vi "Tosca-Plot AI Data.vi"(0 "state in":T2, 5 "Data":cluster{dbl[][], "DI":bool[][]}, 11 "error in (no error)":errorcluster, 12 "Analog":refnum<vi>, 13 "Controls":T1) -> (4 "state out":T2, 15 "error out":errorcluster)   [LabVIEW 2020]
uses:
  Typedefs/Tosca-AI Plot State.ctl
  Typedefs/Tosca-AI Live Controls.ctl
  epl-vi-lib/Utility VIs/Array Manipulation VIs/Array-Dimensions (2D).vi
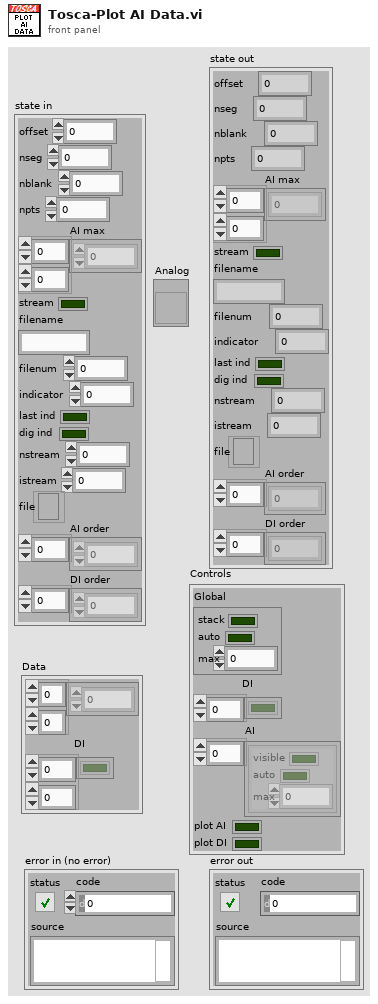
[diagram p1: front panel]
types:
  T1 = typedef "Tosca-AI Live Controls.ctl" = cluster{"Global":cluster{"stack":bool, "auto":bool, "max":dbl}, "DI":bool[], "AI":cluster{"visible":bool, "auto":bool, "max":dbl}[], "plot AI":bool, "plot DI":bool}
  T2 = typedef "Tosca-AI Plot State.ctl" = cluster{"offset":i32, "nseg":i32, "nblank":i32, "npts":i32, "AI max":dbl[][], "stream":bool, "filename":string, "filenum":i32, "indicator":i32, "last ind":bool, "dig ind":bool, "nstream":i32, "istream":i32, "file":refnum<file>, "AI order":i32[], "DI order":i32[]}
  T3 = cluster{"visible":bool, "auto":bool, "max":dbl}[]
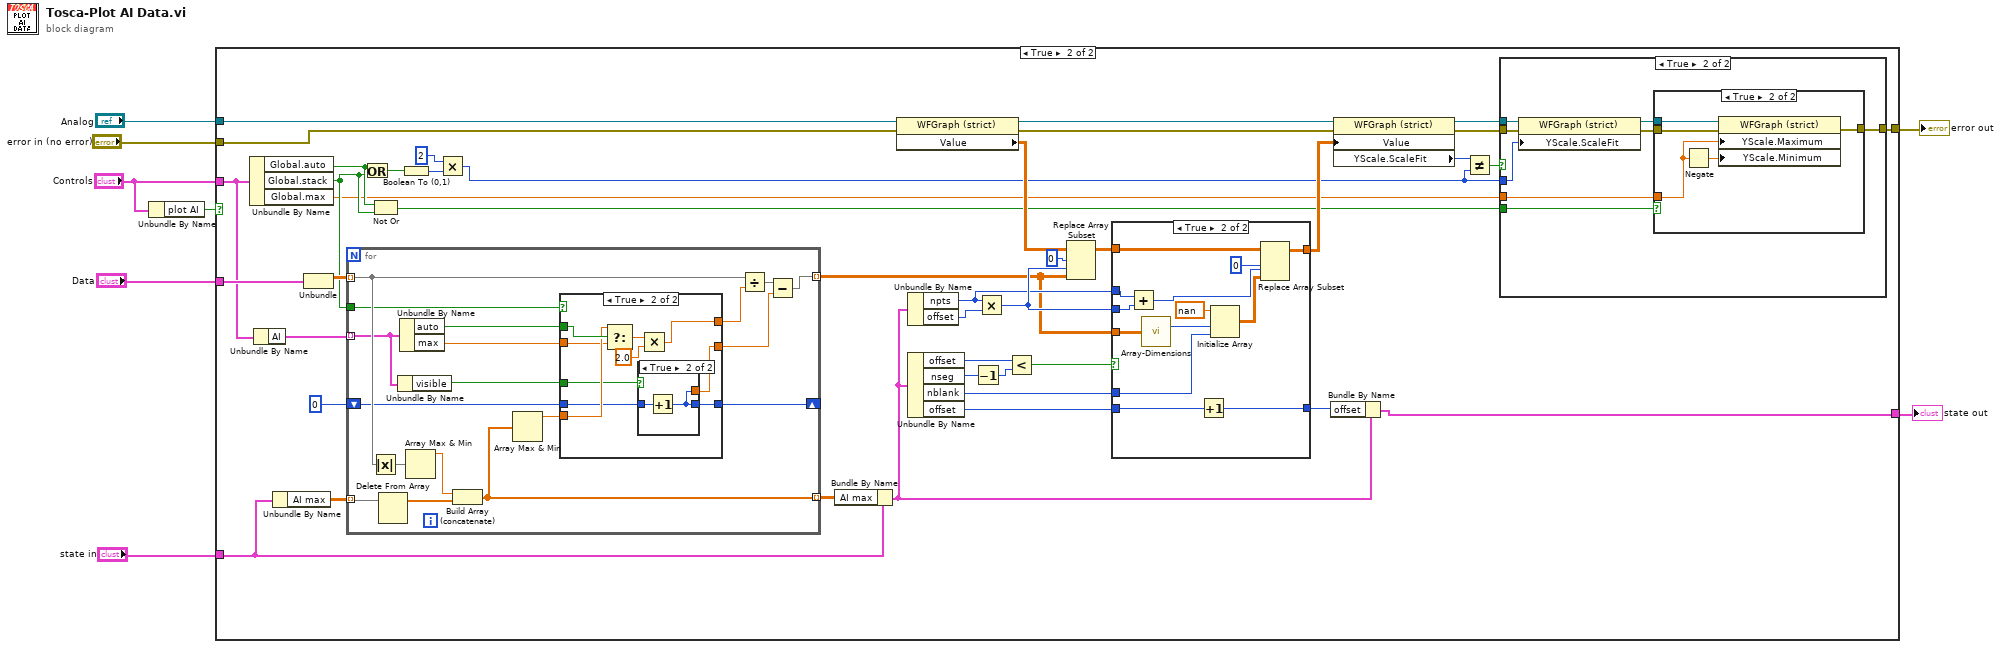
[diagram p0: block diagram]
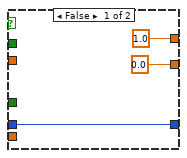
[diagram p5: hidden frame]
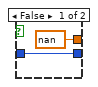
[diagram p6: hidden frame]
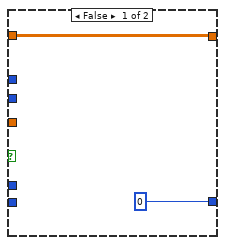
[diagram p7: hidden frame]
diagram:
  n1 = Unbundle By Name("Controls") -> ("plot AI"=w2:bool)
  n2 = case shown="True" w2 {
    tunnel: "Analog" -> [_ w52]
    tunnel: "error in (no error)" -> [w10 w51]
    tunnel: "Data" -> [_ w50]
    tunnel: "state in" -> [w9 w31]
    tunnel: "Controls" -> [_ w26]
    tunnel: [w10 w14] -> w4
    tunnel: [w9 w11] -> w1
    frame False {
    }
    frame True {
      n3 = Unbundle By Name(w26) -> ("Global.auto"=w21:bool, "Global.stack"=w20:bool, "Global.max"=w12:dbl)
      n4 = Unbundle By Name(w26) -> ("AI"=w27:T3)
      n5 = Unbundle By Name(w31) -> ("AI max"=w30:dbl[][])
      n6 = Unbundle(w50) -> (w33:dbl[][])  [unwired: 1 out]
      n7 = for {
        tunnel: w33 -> [w84] mode=indexing
        tunnel: [w85] -> w32 mode=indexing
        tunnel: w30 -> [w82] mode=indexing
        tunnel: [w78] -> w28 mode=indexing
        tunnel: w20 -> [w75]
        tunnel: w27 -> [w69] mode=indexing
        shift-right: [w76] -> _
        shift-left: 0 -> [w77]
        n8 = Absolute Value(x=w84) -> (abs(x)=w83:dbl[])
        n9 = Delete From Array(array=w82) -> (array with subset deleted=w80:dbl[])  [unwired: 2 in, 1 out]
        n10 = Unbundle By Name(w69) -> ("visible"=w68:bool)
        n11 = Unbundle By Name(w69) -> ("auto"=w72:bool, "max"=w70:dbl)
        n12 = Array Max & Min(array=w83) -> (max value=w79:dbl)  [unwired: 3 out]
        n13 = Build Array (concatenate)(w79, w80) -> (w78:dbl[])
        n14 = Array Max & Min(array=w78) -> (max value=w71:dbl)  [unwired: 3 out]
        n15 = case shown="True" w75 {
          tunnel: w77 -> [w87 w91]
          tunnel: [w87 w90] -> w76
          tunnel: [1.0 w93] -> w74
          tunnel: [0.0 w89] -> w73
          tunnel: w72 -> [_ w98]
          tunnel: w71 -> [_ w97]
          tunnel: w70 -> [_ w96]
          tunnel: w68 -> [_ w92]
          frame False {
          }
          frame True {
            n16 = Select(t=w97, s=w98, f=w96) -> (s? t:f=w95:dbl)
            n17 = case shown="True" w92 {
              tunnel: w91 -> [w100 w102]
              tunnel: [w100 w101] -> w90
              tunnel: [nan w101] -> w89
              frame False {
              }
              frame True {
                n18 = Increment(x=w102) -> (x+1=w101:i32)
              }
            }
            n19 = Multiply(x=w95, y=2.0) -> (x*y=w93:dbl)
          }
        }
        n20 = Divide(x=w84, y=w74) -> (x/y=w81:dbl[])
        n21 = Subtract(x=w81, y=w73) -> (x-y=w85:dbl[])
      }
      n22 = Or(x=w21, y=w20) -> (x .or. y?=w25:bool)
      n23 = Not Or(1:w20, 2:w21) -> (0:w13:bool)
      n24 = Boolean To (0,1)(Boolean=w25) -> (0, 1=w24:i16)
      n25 = Multiply(x=i16 2 ("y"), y=w24) -> (x*y=w15:i16)
      n26 = Bundle By Name(cluster=w31, "AI max"=w28) -> (w29:T2)
      n27 = property class="WFGraph (strict)"(reference=w52, error in=w51) -> (reference out=w47:refnum<vi>, error out=w46:errorcluster, "Value"=w49:dbl[][])
      n28 = Unbundle By Name(w29) -> ("npts"=w37:i32, "offset"=w45:i32)
      n29 = Unbundle By Name(w29) -> ("offset"=w44:i32, "nseg"=w43:i32, "nblank"=w41:i32, "offset"=w35:i32)
      n30 = Decrement(x=w43) -> (x-1=w42:i32)
      n31 = Multiply(x=w37, y=w45) -> (x*y=w38:i32)
      n32 = Less?(x=w44, y=w42) -> (x < y?=w39:bool)
      n33 = Replace Array Subset(array=w49, new element=w32, index (row)=0 ("disabled index (row)"), index (col)=w38) -> (w40:dbl[][])
      n34 = case shown="True" w39 {
        tunnel: w32 -> [_ w117]
        tunnel: w41 -> [_ w115]
        tunnel: w40 -> [w104 w113]
        tunnel: w38 -> [_ w110]
        tunnel: w37 -> [_ w109]
        tunnel: [w104 w107] -> w36
        tunnel: w35 -> [_ w106]
        tunnel: [0 w105] -> w34
        frame False {
        }
        frame True {
          n35 = Add(x=w109, y=w110) -> (x+y=w108:i32)
          n36 = call-poly "Array-Dimensions.vi"("2D Array"=w117) -> ("# rows"=w116:i32)  [unwired: 13 in, 1 out]
          n37 = Increment(x=w106) -> (x+1=w105:i32)
          n38 = Initialize Array(nan, w116, w115) -> (w112:dbl[][])
          n39 = Replace Array Subset(array=w113, new element=w112, index (row)=0, index (col)=w108) -> (w107:dbl[][])
        }
      }
      n40 = Bundle By Name(cluster=w29, "offset"=w34) -> (w11:T2)
      n41 = property class="WFGraph (strict)"(reference=w47, error in=w46, "Value"=w36) -> (reference out=w19:refnum<vi>, error out=w18:errorcluster, "YScale.ScaleFit"=w17:u8)
      n42 = Not Equal?(x=w17, y=w15) -> (x != y?=w16:bool)
      n43 = case shown="True" w16 {
        tunnel: w19 -> [_ w61]
        tunnel: [w53 w56] -> w14
        tunnel: w18 -> [w53 w60]
        tunnel: w15 -> [_ w59]
        tunnel: w13 -> [_ w55]
        tunnel: w12 -> [_ w54]
        frame False {
        }
        frame True {
          n44 = property class="WFGraph (strict)"(reference=w61, error in=w60, "YScale.ScaleFit"=w59) -> (reference out=w58:refnum<vi>, error out=w57:errorcluster)
          n45 = case shown="True" w55 {
            tunnel: w58 -> [_ w67]
            tunnel: w57 -> [w62 w66]
            tunnel: [w62 w65] -> w56
            tunnel: w54 -> [_ w63]
            frame False {
            }
            frame True {
              n46 = Negate(x=w63) -> (-x=w64:dbl)
              n47 = property class="WFGraph (strict)"(reference=w67, error in=w66, "YScale.Maximum"=w63, "YScale.Minimum"=w64) -> (error out=w65:errorcluster)  [unwired: 1 out]
            }
          }
        }
      }
    }
  }
  "error out" <- w4
  "state out" <- w1
